vi "Exemple - AsyncRepeatSum.vi"() -> ()   [LabVIEW 2016]
uses:
  Library/DemoSkeleton/DemoSkeleton.lvlib
panel:
  in  "stop":bool
  in  "B":i32=2
  in  "A":i32=1
  out "Sum":i64
  # "+"
  # "="
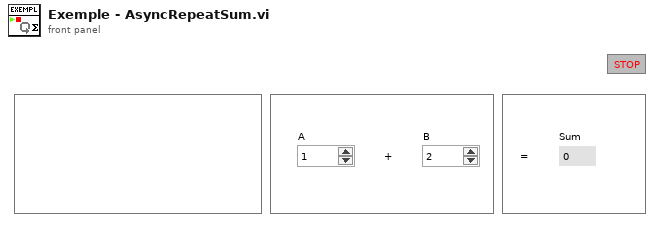
[diagram p1: front panel]
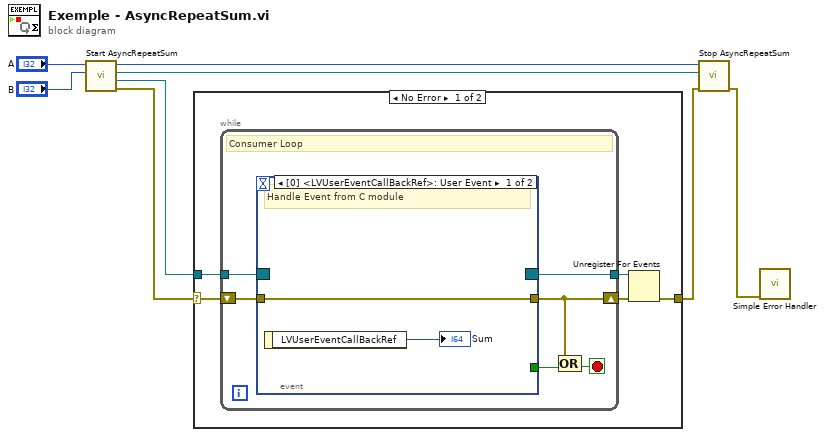
[diagram p0: block diagram]
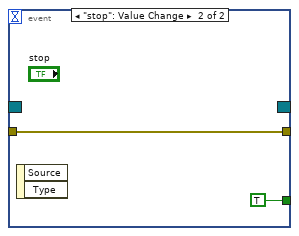
[diagram p2: hidden frame]
diagram:
  n1 = call "Start AsyncRepeatSum.vi"("B"="B", "A"="A") -> ("error out"=w6:errorcluster, "AsyncSum Event Register"=w5:refnum<event-registration>, "LVUserEvent CallBack Reference"=w3:refnum<user-event>, "Handle"=w4:u64)  [unwired: 6 in]
  n2 = case shown="No Error" w6 {
    selector: w6 -> [w11 w24]
    tunnel: w5 -> [w10 _]
    tunnel: [w9 w24] -> w2
    frame No Error {
      n3 = while {
        shift-right: [w16] -> w12
        shift-left: w11 -> [w18]
        tunnel: w10 -> [w17]
        tunnel: [w19] -> w13
        stop <- w15 stop-if-true
        # "Consumer Loop"
        n4 = event shown="[0] <LVUserEventCallBackRef>: User Event" {
          selector: w17 -> [_ _]
          dyn-events: [_ _] -> w19
          timeout: _ -> [_ _]
          tunnel: w18 -> [w21 w23]
          tunnel: [w21 w23] -> w16
          tunnel: [_ TRUE] -> w14
          event User Event {
            # "Handle Event from C module"
            n5 = event-data() -> ("LVUserEventCallBackRef"=→"Sum":i64)  [unwired: 1 in]
          }
          event "stop": Value Change {
            n6 = event-data() -> ()  [unwired: 1 in, 2 out]
          }
        }
        n7 = Compound Arithmetic op=OR(w16, w14) -> (w15:bool)
      }
      n8 = Unregister For Events(event registration refnum=w13, error in=w12) -> (error out=w9:errorcluster)
    }
    frame Error {
    }
  }
  n9 = call "Stop AsyncRepeatSum.vi"("error in (no error)"=w2, "LVUserEventCallBackRef"=w3, "Handle"=w4) -> ("error out"=w1:errorcluster)  [unwired: 8 in]
  n10 = call <vilib>:"Simple Error Handler.vi"("error in (no error)"=w1) -> ()  [unwired: 4 in, 5 out]
